vi "Stop Core.vi"(10 "final error code":i32, 11 "MusicManagerActor in":refnum<class "MusicManagerActor.lvclass">) -> (3 "MusicManagerActor out":refnum<class "MusicManagerActor.lvclass">)   [LabVIEW 2015, in "MusicManagerActor.lvlib" / "MusicManagerActor.lvclass"]
doc: "(<B>Filename</B>: Actor Framework.lvlib:Actor.lvclass:Stop Core.vi)\n\nDefines what the actor does before it stops. Use the <B>final error code</B> input to determine whether the actor shut down in response to an error.\n\nBy default, this method does nothing. A descendant class may override it to define behavior, such as shutting down any processes the actor initiated in its override of the Actor Core method."
uses:
  MusicManagerActor.lvclass
  MusicManagerActor.lvclass/MusicManagerActor.ctl
  <vilib>/ActorFramework/Actor/Actor.lvclass
  config/App Config/App Config.lvlib
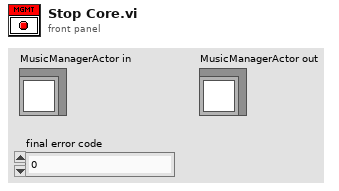
[diagram p1: front panel]
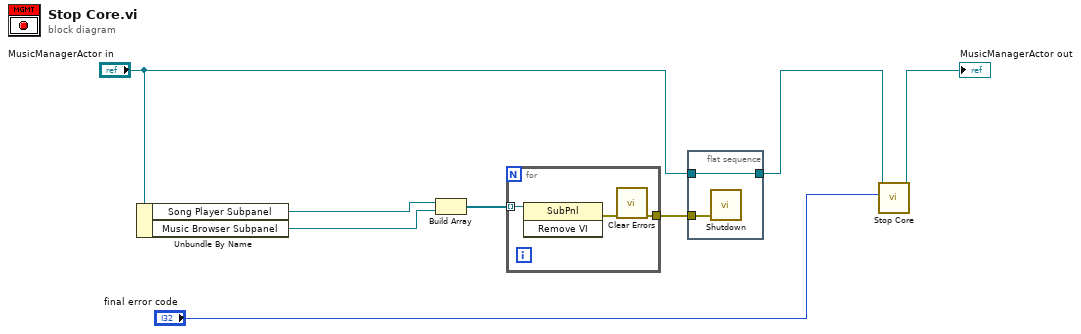
[diagram p0: block diagram]
diagram:
  n1 = Unbundle By Name("MusicManagerActor in") -> ("Song Player Subpanel"=w3:refnum<vi>, "Music Browser Subpanel"=w2:refnum<vi>)
  n2 = Build Array(w3, w2) -> (w6:refnum<vi>[])
  n3 = for {
    tunnel: w6 -> [w10] mode=indexing
    tunnel: [w9] -> w5
    n4 = invoke class="SubPnl" method="Remove VI"(reference=w10) -> (error out=w11:errorcluster)  [unwired: 2 in, 2 out]
    n5 = call <vilib>:"Clear Errors.vi"("error in (no error)"=w11) -> ("error out"=w9:errorcluster)  [unwired: 5 in, 1 out]
  }
  n6 = flat-sequence {
    tunnel: w5 -> [w13]
    tunnel: "MusicManagerActor in" -> [w12]
    tunnel: [w12] -> w4
    frame #0 {
      n7 = call "Shutdown.vi"("error in (no error)"=w13) -> ()  [unwired: 10 in, 1 out]
    }
  }
  n8 = call-parent "Stop Core.vi"("final error code"="final error code", "Actor in"=w4) -> ("Actor out"=→"MusicManagerActor out":refnum<class "MusicManagerActor.lvclass">)  [unwired: 9 in]
